vi "GetDistance.vi"(8 "Target Height (h2)":dbl, 9 "Camera Height (h1)":dbl, 10 "Camera-Target Angle (a2)":dbl, 11 "Camera-Ground Angle (a1)":dbl) -> (2 "Distance  to Target":dbl)   [LabVIEW 2019]
panel:
  # "Usually Limelight's Y offset"
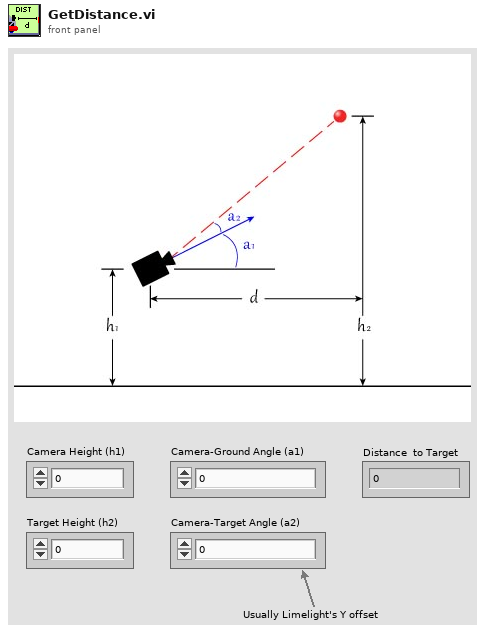
[diagram p1: front panel]
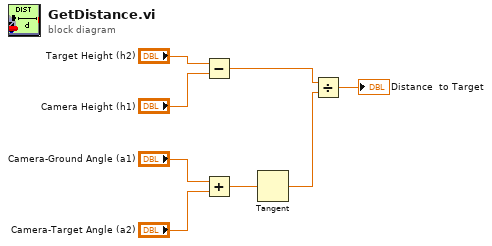
[diagram p0: block diagram]
diagram:
  n1 = Subtract(x="Target Height (h2)", y="Camera Height (h1)") -> (x-y=w6:dbl)
  n2 = Add(x="Camera-Ground Angle (a1)", y="Camera-Target Angle (a2)") -> (x+y=w3:dbl)
  n3 = Tangent(1:w3) -> (0:w2:dbl)
  n4 = Divide(x=w6, y=w2) -> (x/y=→"Distance  to Target":dbl)
